vi "Read shared registers.vi"(8 "error in (no error)":errorcluster, 11 "niUSRP Rx Core v1 FPGA in":refnum<class "niUSRP Sync v1 FPGA.lvclass">) -> (0 "error out":errorcluster, 2 "niInstr Instruction Framework Interfaces v1 FPGA.lvlib:Address Space Collection.lvclass":refnum<class "Address Space Collection.lvclass">, 3 "niUSRP Rx Core v1 FPGA out":refnum<class "niUSRP Sync v1 FPGA.lvclass">)   [LabVIEW 2025, in "niUSRP Sync v1 FPGA.lvclass"]
uses:
  niUSRP Sync v1 FPGA.lvclass
  <instrlib>/_niInstr/Instruction Framework/v1/FPGA/Interfaces/Address Space Collection/Address Space Collection.lvclass
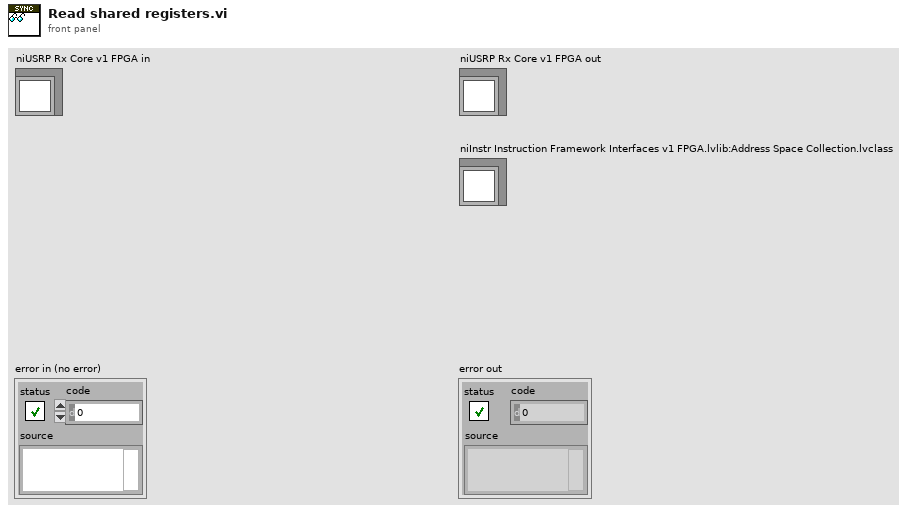
[diagram p1: front panel]
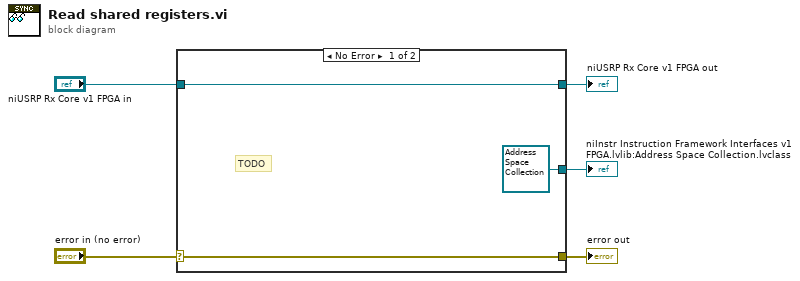
[diagram p0: block diagram]
diagram:
  n1 = case shown="No Error" "error in (no error)" {
    selector: "error in (no error)" -> [w8 w9]
    tunnel: [w8 w9] -> w4
    tunnel: [w7 w10] -> w2
    tunnel: "niUSRP Rx Core v1 FPGA in" -> [w7 w10]
    tunnel: [refnum<class "Address Space Collection.lvclass"> refnum ("shared registers") _] -> w1
    frame No Error {
      # "TODO"
    }
    frame Error {
    }
  }
  "error out" <- w4
  "niUSRP Rx Core v1 FPGA out" <- w2
  "niInstr Instruction Framework Interfaces v1 FPGA.lvlib:Address Space Collection.lvclass" <- w1
